vi "strobe_digital_in.vi"() -> ()   [LabVIEW 2016]
panel:
  out "Stim ID":dbl
  out "StimTrigger":bool
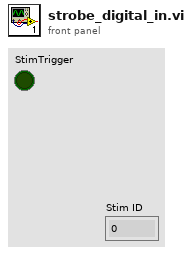
[diagram p1: front panel]
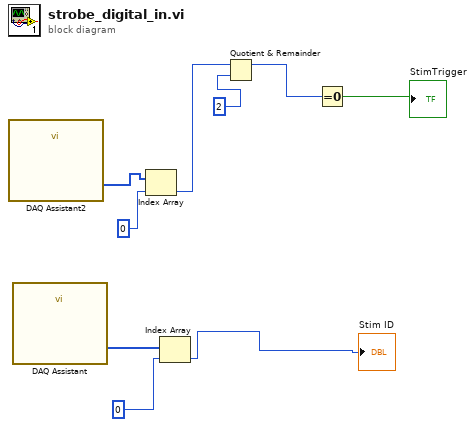
[diagram p0: block diagram]
diagram:
  n1 = call "DAQ Assistant2"() -> ("data"=w6:u32[])  [unwired: 17 in, 2 out]
  n2 = call "DAQ Assistant"() -> ("data"=w8:u32[])  [unwired: 17 in, 2 out]
  n3 = Index Array(array=w6, index=0) -> (element=w4:u32)
  n4 = Index Array(array=w8, index=0) -> (element=→"Stim ID":u32)
  n5 = Quotient & Remainder(x=w4, y=2) -> (x-y*floor(x/y)=w2:u32)  [unwired: 1 out]
  n6 = Equal To 0?(x=w2) -> (x = 0?=→"StimTrigger":bool)
